vi "SE Mask Offset Outer List Configure Offset Freq Def.vi"(8 "error in (no error)":errorcluster {"code" format="%.0x"}, 9 "OffsetFrequencyDefine (Inner Offset Frequency Definitioncto Center)":i32(ring) items=["Inner Offset Frequency Definitioncto Center", "Inner Offset Frequency Definitioncto Edge", "Inner Offset Frequency Definitioneto Center", "Inner Offset Frequency Definitioneto Edge"], 11 "instrument handle":refnum<k15>) -> (0 "error out":errorcluster {"code" format="%.0x"}, 3 "instrument handle out":refnum<k15>)   [LabVIEW 2021, in "Keysight XSAnVMA.lvlib"]
doc: "This method allows to select 'Offset' definition. Each standard defines each 'Offset' from Carrier."
uses:
  <instrlib>/Keysight XSAnVMA/Keysight XSAnVMA.lvlib
  KtXSAnVMA_64.dll
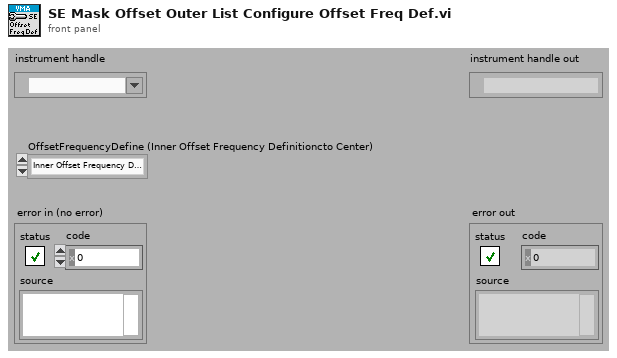
[diagram p1: front panel]
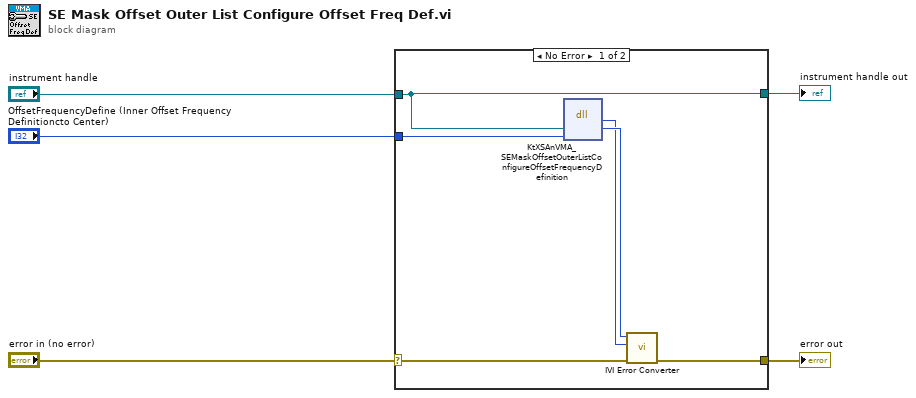
[diagram p0: block diagram]
diagram:
  n1 = case shown="No Error" "error in (no error)" {
    selector: "error in (no error)" -> [w9 w13]
    tunnel: [w8 w13] -> w5
    tunnel: "instrument handle" -> [w6 w12]
    tunnel: "OffsetFrequencyDefine (Inner Offset Frequency Definitioncto Center)" -> [w7 _]
    tunnel: [w6 w12] -> w1
    frame No Error {
      n2 = dll-call lib="KtXSAnVMA**.dll" fn="KtXSAnVMA_SEMaskOffsetOuterListConfigureOffsetFrequencyDefinition"("Vi"=w6, "OffsetFrequencyDefine"=w7) -> (w10:i32, "Vi"=w11:u32)  [unwired: 4 in, 2 out]
      n3 = call <instrlib>:"IVI Error Converter.vi"("error in (no error)"=w9, "IVI error code (0)"=w10, "instrument handle"=w11) -> ("error out"=w8:errorcluster)  [unwired: 7 in, 1 out]
    }
    frame Error {
    }
  }
  "error out" <- w5
  "instrument handle out" <- w1
